vi "NI VeriStand - Get Timed Loop Priority.vi"(8 "error in (no error)":errorcluster, 11 "Device Ref in":T2 format="%.0x") -> (0 "error out":errorcluster, 2 "Priority":T1, 3 "Device Ref out":T2 format="%.0x")   [LabVIEW 2020, in "Custom Device API.lvlib"]
doc: "Returns the priority (<B>Low</B>, <B>Medium</B>, or <B>High</B>) of an asynchronous custom device Timed Loop. To convert this enumerated value to a numeric value that the Timed Loop input terminal accepts, use the NI VeriStand - Convert Timed Loop Priority Property to Number VI."
uses:
  <vilib>/NI VeriStand/Custom Device API/Custom Device API.lvlib
  <vilib>/NI VeriStand/Custom Device API/Custom Device Item Ref.ctl
  <vilib>/NI VeriStand/Custom Device API/Custom Device Timed Loop Priority.ctl
  6675235e-156f-4b79-9c1d-11b99208b075.vi
  <vilib>/NI VeriStand/Custom Device API/Custom Device Offline Path.vi
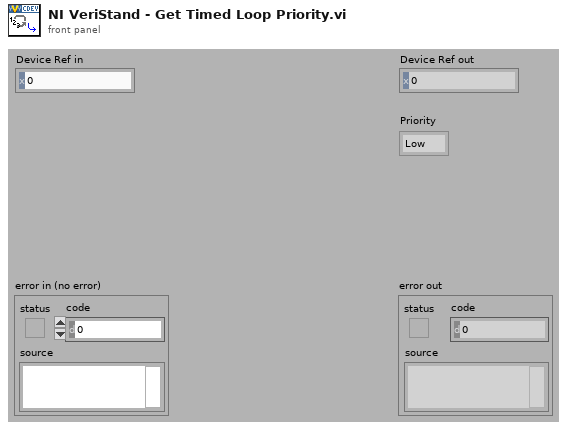
[diagram p1: front panel]
types:
  T1 = typedef "Custom Device API.lvlib/Custom Device Timed Loop Priority.ctl" = enum32{"Low", "Medium", "High"}
  T2 = typedef "Custom Device API.lvlib/Custom Device Item Ref.ctl" = u64
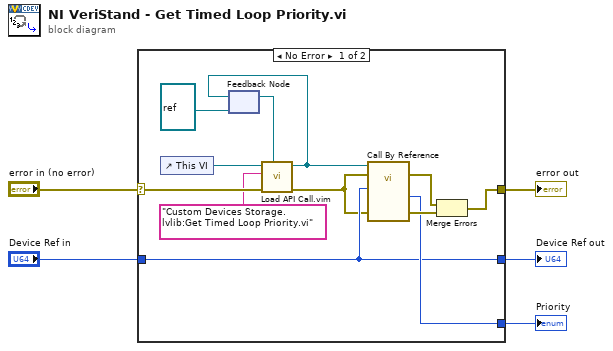
[diagram p0: block diagram]
diagram:
  n1 = case shown="No Error" "error in (no error)" {
    selector: "error in (no error)" -> [w11 w18]
    tunnel: [w16 w18] -> w5
    tunnel: "Device Ref in" -> [w14 w19]
    tunnel: [w14 w19] -> w3
    tunnel: [w15 _] -> w2
    frame No Error {
      n2 = control-ref of="This VI"() -> (w12:refnum<vi>)
      n3 = feedback #1(refnum<vi> refnum ("type specifier VI Refnum (for type only)")) -> (w13:refnum<vi>)
      n4 = call "Load API Call.vim"("VI reference in"=w13, "error in (no error)"=w11, "VI qualified name"="Custom Devices Storage.lvlib:Get Timed Loop Priority.vi", "Caller VI ref"=w12) -> ("error out"=w10:errorcluster, "VI reference"=w9:refnum<vi>)  [unwired: 6 in]
      n5 = feedback-in #1(w9) -> ()
      n6 = call-by-ref "?"(reference=w9, error in=w10, 8:"error in (no error)"=w10, "Device Ref in"=w14) -> (error out=w6:errorcluster, 0:"error out"=w17:errorcluster, "Priority"=w15:T1)  [unwired: 7 in, 2 out]
      n7 = Merge Errors(w6, w17) -> (w16:errorcluster)
    }
    frame Error {
    }
  }
  "Device Ref out" <- w3
  "error out" <- w5
  "Priority" <- w2
